vi "control plot scale V1.vi"(6 "offset in":dbl=nan, 7 "action":T2(ring), 8 "Coords":T3, 9 "fraction in":dbl, 11 "plot scale state":T1={"Plot Ref"=refnum, "center"=0.0, "delta"=100.0, "mode"=enum."no filter", "scale cursor index"=0, "history"=100.0, "history array"=[0.5, 0.5, 0.5, 0.5, 0.5, 0.5, 0.5, 0.5, 0.5, 0.5, 0.5, 0.5, 0.5, 0.5, 0.5, 0.5, 0.5, 0.5, 0.5, 0.5, 0.5, 0.5, 0.5, 0.5, 0.5, 0.5, 0.5, 0.5, 0.5, 0.5, 0.5, 0.5, 0.5, 0.5, 0.5, 0.5, 0.5, 0.5, 0.5, 0.5, 0.5, 0.5, 0.5, 0.5, 0.5, 0.5, 0.5, 0.5, 0.5, 0.5, 0.5, 0.5, 0.5, 0.5, 0.5, 0.5, 0.5, 0.5, 0.5, 0.5, 0.5, 0.5, 0.5, 0.5, 0.5, 0.5, 0.5, 0.5, 0.5, 0.5, 0.5, 0.5, 0.5, 0.5, 0.5, 0.5, 0.5, 0.5, 0.5, 0.5, 0.5, 0.5, 0.5, 0.5, 0.5, 0.5, 0.5, 0.5, 0.5, 0.5, 0.5, 0.5, 0.5, 0.5, 0.5, 0.5, 0.5, 0.5, 0.5, 0.5]}) -> (1 "fraction out":dbl, 3 "plot scale state out":T1={"Plot Ref"=refnum, "center"=0.0, "delta"=100.0, "mode"=enum."no filter", "scale cursor index"=0, "history"=100.0, "history array"=[0.5, 0.5, 0.5, 0.5, 0.5, 0.5, 0.5, 0.5, 0.5, 0.5, 0.5, 0.5, 0.5, 0.5, 0.5, 0.5, 0.5, 0.5, 0.5, 0.5, 0.5, 0.5, 0.5, 0.5, 0.5, 0.5, 0.5, 0.5, 0.5, 0.5, 0.5, 0.5, 0.5, 0.5, 0.5, 0.5, 0.5, 0.5, 0.5, 0.5, 0.5, 0.5, 0.5, 0.5, 0.5, 0.5, 0.5, 0.5, 0.5, 0.5, 0.5, 0.5, 0.5, 0.5, 0.5, 0.5, 0.5, 0.5, 0.5, 0.5, 0.5, 0.5, 0.5, 0.5, 0.5, 0.5, 0.5, 0.5, 0.5, 0.5, 0.5, 0.5, 0.5, 0.5, 0.5, 0.5, 0.5, 0.5, 0.5, 0.5, 0.5, 0.5, 0.5, 0.5, 0.5, 0.5, 0.5, 0.5, 0.5, 0.5, 0.5, 0.5, 0.5, 0.5, 0.5, 0.5, 0.5, 0.5, 0.5, 0.5]})   [LabVIEW 2015]
uses:
  <vilib>/Utility/miscctls.llb/LVPoint32TypeDef.ctl
  plot scale state.ctl
  <vilib>/Analysis/6fits.llb/Curve Fitting Criteria.ctl
  <vilib>/Analysis/NI_AALPro.lvlib
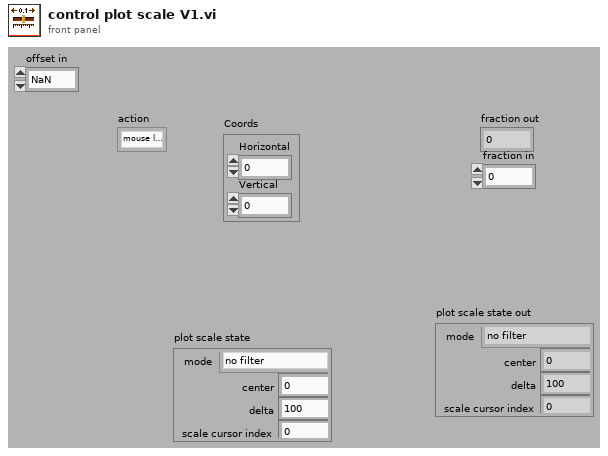
[diagram p1: front panel]
types:
  T1 = typedef "plot scale state.ctl" = cluster{"Plot Ref":refnum<vi>, "center":dbl, "delta":dbl, "mode":enum16{"no filter", "median", "liner fit on median"}, "scale cursor index":i32, "history":dbl, "history array":dbl[]}
  T2 = enum16{"mouse leave", "mouse enter", "mouse move", "manual zoom both", "manual zoom x", "manual zoom y"}
  T3 = typedef "LVPoint32TypeDef.ctl" = cluster{"Horizontal":i32, "Vertical":i32}
  T4 = typedef "LVCursorListTypeDef.ctl" = cluster{"Name":string, "Color":u32, "Style":u8, "Point Style":u8, "Name Visible":bool, "Allow Drag":bool, "Cursor Mode":u32, "Plot":i32, "Index":i32, "Position":cluster{"X":dbl, "Y":dbl}, "X Scale":u32, "Y Scale":u32, "Watch Plots":i32[], "Watch All Plots":bool, "Plot Area":i32, "Label Offset":cluster{"X":dbl, "Y":dbl}}[]
  T5 = cluster{"Name":string, "Color":u32, "Style":u8, "Point Style":u8, "Name Visible":bool, "Allow Drag":bool, "Cursor Mode":u32, "Plot":i32, "Index":i32, "Position":cluster{"X":dbl, "Y":dbl}, "X Scale":u32, "Y Scale":u32, "Watch Plots":i32[], "Watch All Plots":bool, "Plot Area":i32, "Label Offset":cluster{"X":dbl, "Y":dbl}}
  T6 = typedef "LVBoundsTypeDef.ctl" = cluster{"Width":u32, "Height":u32}
  T7 = typedef "LVPositionTypeDef.ctl" = cluster{"Left":i32, "Top":i32}
  T8 = typedef "NI_AALPro.lvlib/Curve Fitting Criteria.ctl" = u16
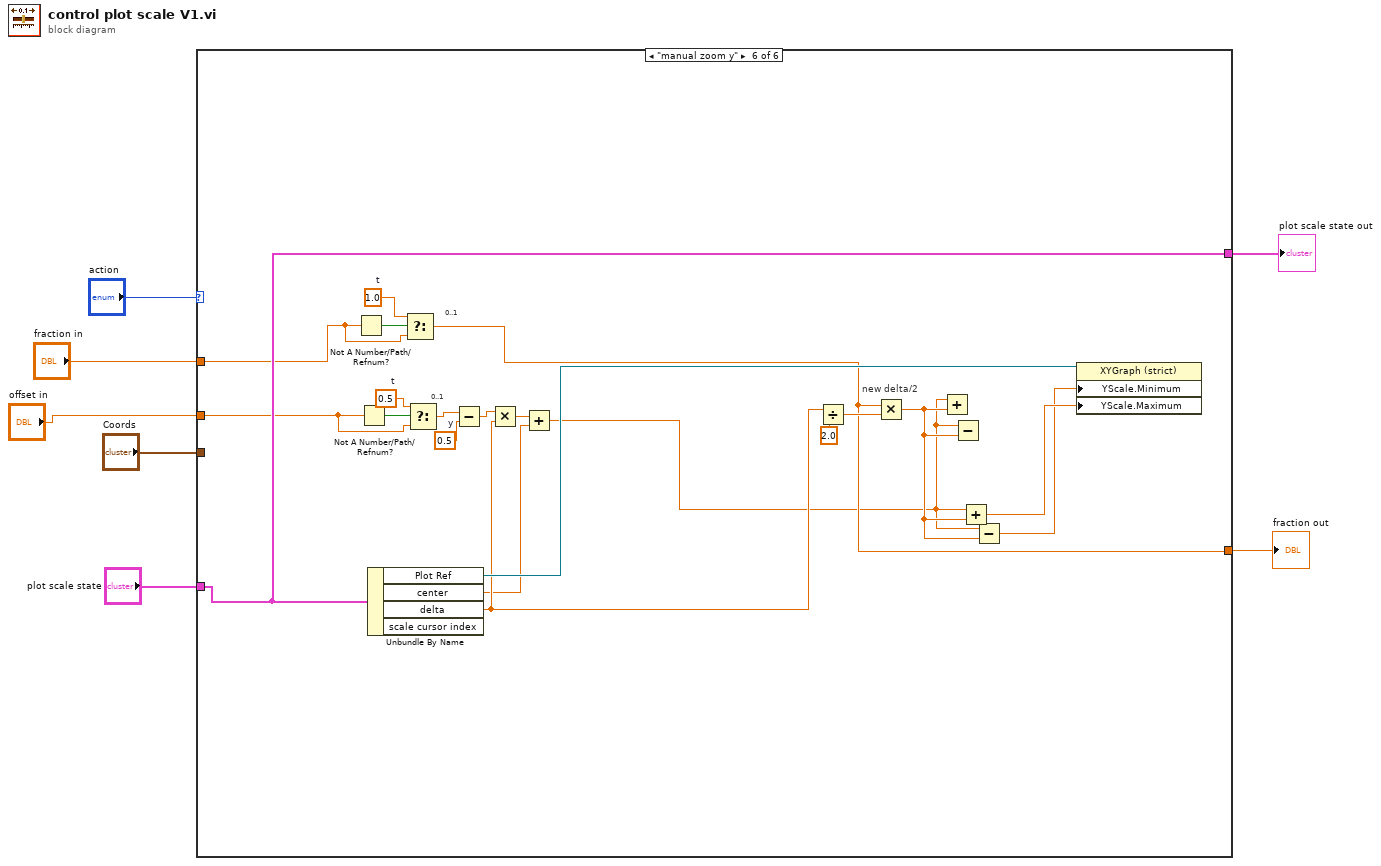
[diagram p0: block diagram]
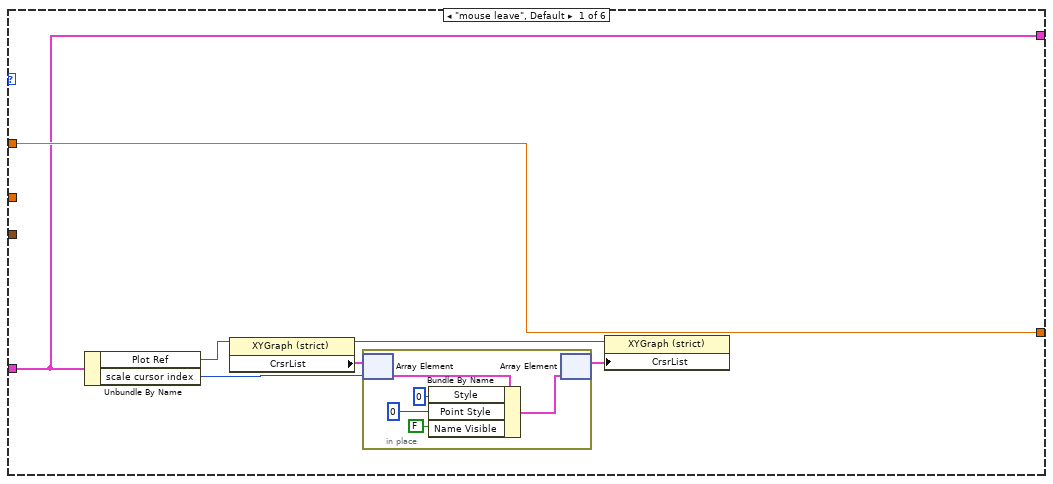
[diagram p2: hidden frame]
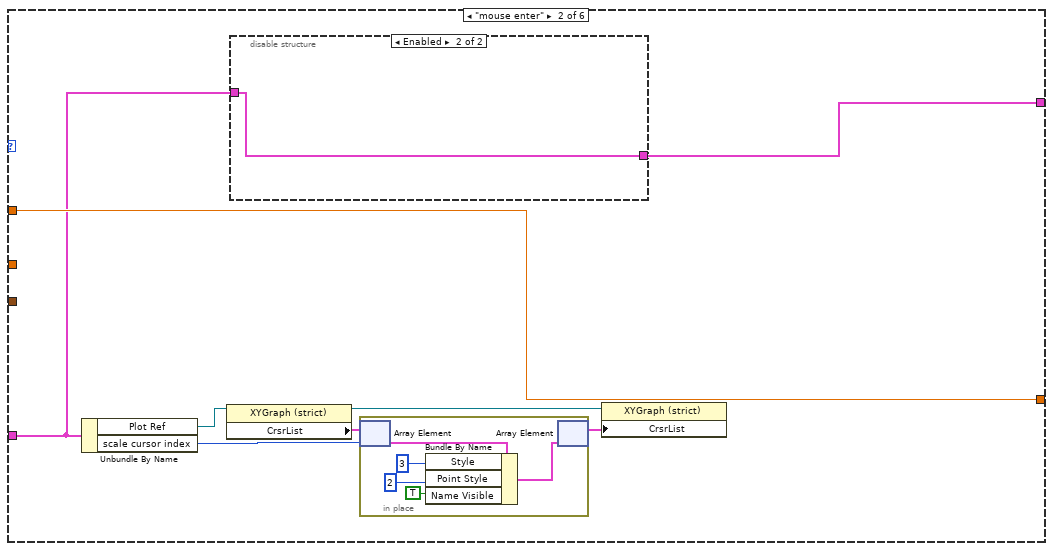
[diagram p3: hidden frame]
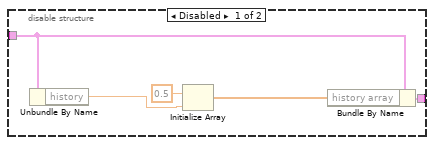
[diagram p4: hidden frame]
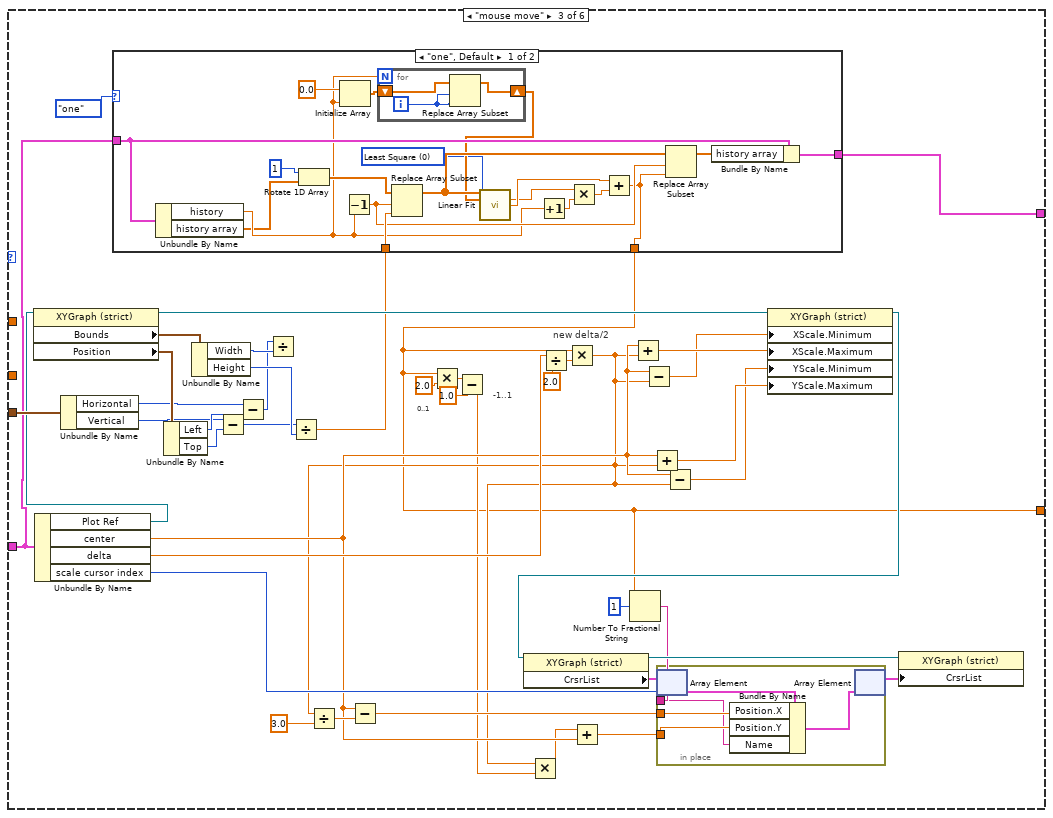
[diagram p5: hidden frame]
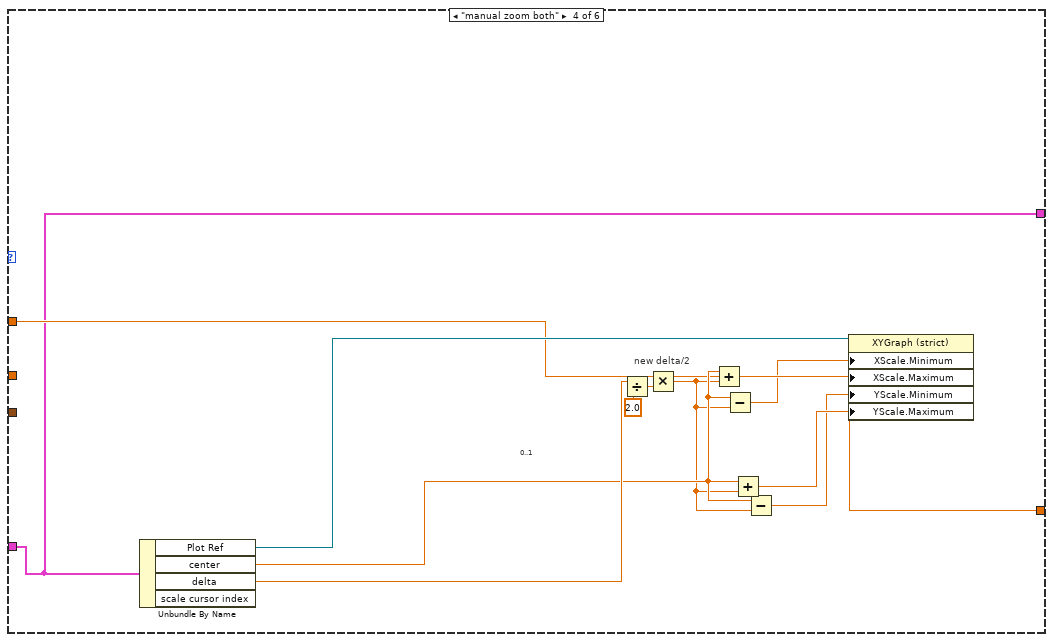
[diagram p7: hidden frame]
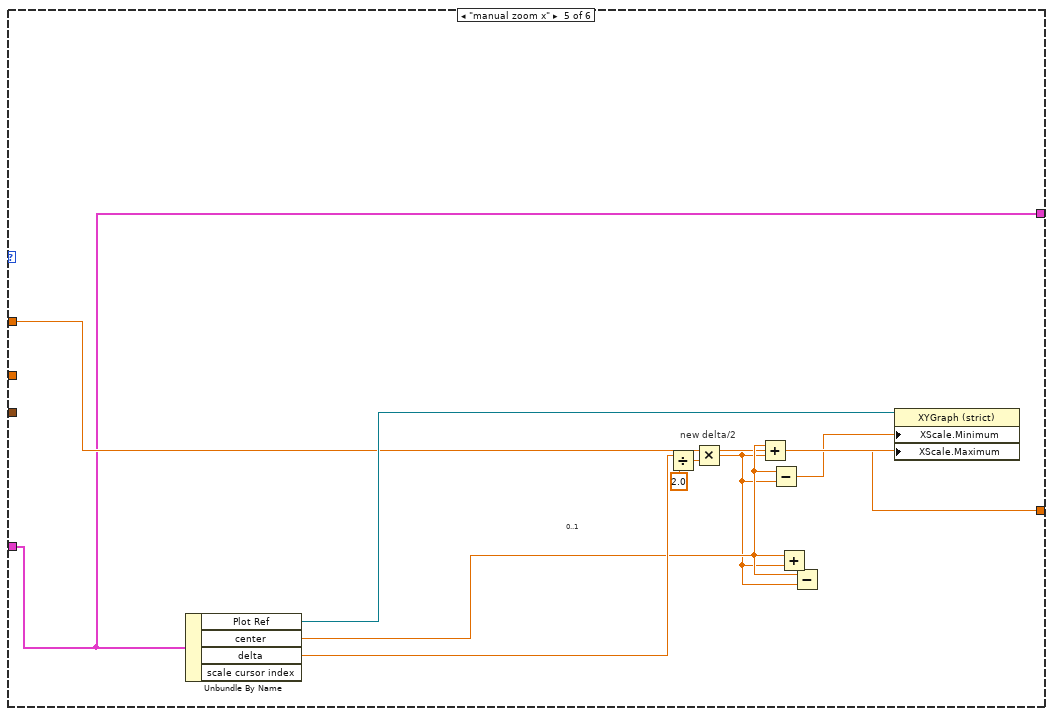
[diagram p8: hidden frame]
diagram:
  n1 = case shown="\"manual zoom y\"" "action" {
    tunnel: "Coords" -> [_ _ w64 _ _ _]
    tunnel: "plot scale state" -> [w8 w21 w43 w111 w123 w147]
    tunnel: [w9 w22 w40 w112 w124 w141] -> w4
    tunnel: "fraction in" -> [w9 w22 _ w112 w124 w142]
    tunnel: [w8 w20 w42 w111 w123 w147] -> w2
    tunnel: "offset in" -> [_ _ _ _ _ w145]
    frame "mouse leave", Default {
      n2 = Unbundle By Name(w8) -> ("Plot Ref"=w14:refnum<vi>, "scale cursor index"=w12:i32)
      n3 = property on="Property Node" class="XYGraph (strict)"(reference=w14) -> (reference out=w10:refnum<vi>, "CrsrList"=w13:T4)  [unwired: 1 in, 1 out]
      n4 = in-place {
        n5 = in-place-array #1(w13, w12) -> (w19:T5)
        n6 = Bundle By Name(cluster=w19, "Style"=u8 0, "Point Style"=u8 0, "Name Visible"=FALSE) -> (w18:T5)
        n7 = in-place-array #1(w18) -> (w11:T4)  [unwired: 1 out]
      }
      n8 = property on="Property Node" class="XYGraph (strict)"(reference=w10, "CrsrList"=w11) -> ()  [unwired: 1 in, 2 out]
    }
    frame "mouse enter" {
      n9 = Unbundle By Name(w21) -> ("Plot Ref"=w27:refnum<vi>, "scale cursor index"=w25:i32)
      n10 = property on="Property Node" class="XYGraph (strict)"(reference=w27) -> (reference out=w23:refnum<vi>, "CrsrList"=w26:T4)  [unwired: 1 in, 1 out]
      n11 = disable-structure shown="Enabled" {
        disable-tunnel: w21 -> [w30 w33]
        disable-tunnel: [w29 w33] -> w20
        frame Disabled {
          n12 = Unbundle By Name(w30) -> ("history"=w31:dbl)
          n13 = Initialize Array(0.5 ("element"), w31) -> (w28:dbl[])
          n14 = Bundle By Name(cluster=w30, "history array"=w28) -> (w29:T1)
        }
        frame Enabled {
        }
      }
      n15 = in-place {
        n16 = in-place-array #2(w26, w25) -> (w38:T5)
        n17 = Bundle By Name(cluster=w38, "Style"=u8 3, "Point Style"=u8 2, "Name Visible"=TRUE) -> (w37:T5)
        n18 = in-place-array #2(w37) -> (w24:T4)  [unwired: 1 out]
      }
      n19 = property on="Property Node" class="XYGraph (strict)"(reference=w23, "CrsrList"=w24) -> ()  [unwired: 1 in, 2 out]
    }
    frame "mouse move" {
      # "-1..1"
      # "0..1"
      # "new delta/2"
      n20 = Unbundle By Name(w43) -> ("Plot Ref"=w62:refnum<vi>, "center"=w51:dbl, "delta"=w63:dbl, "scale cursor index"=w58:i32)
      n21 = property on="Property Node" class="XYGraph (strict)"(reference=w62) -> (reference out=w76:refnum<vi>, "Bounds"=w75:T6, "Position"=w81:T7)  [unwired: 1 in, 1 out]
      n22 = Unbundle By Name(w64) -> ("Horizontal"=w80:i32, "Vertical"=w78:i32)
      n23 = Unbundle By Name(w81) -> ("Left"=w79:i32, "Top"=w77:i32)
      n24 = Unbundle By Name(w75) -> ("Width"=w74:u32, "Height"=w73:u32)
      n25 = Subtract(x=w78, y=w77) -> (x-y=w65:i32)
      n26 = Subtract(x=w80, y=w79) -> (x-y=w66:i32)
      n27 = Divide(x=w66, y=w74) -> ()  [unwired: 1 out]
      n28 = Divide(x=w65, y=w73) -> (x/y=w41:dbl)
      n29 = case shown="\"one\", Default" enum16{"one", "two"}."one" {
        tunnel: w43 -> [w88 w105]
        tunnel: [w100 w105] -> w42
        tunnel: w41 -> [w98 w104]
        tunnel: [w82 w104] -> w40
        frame "one", Default {
          w83 = T8 0 items=["Least Square", "Least Absolute Residual", "Bisquare"] ("method")
          n30 = Unbundle By Name(w88) -> ("history"=w87:dbl, "history array"=w86:dbl[])
          n31 = Rotate 1D Array(1:w86, 2:1 ("n")) -> (0:w97:dbl[])
          n32 = Initialize Array(0.0 ("element"), w87) -> (w95:dbl[])
          n33 = Decrement(x=w87) -> (x-1=w89:dbl)
          n34 = for {
            N: w87 -> [_]
            shift-right: [w102] -> w84
            shift-left: w95 -> [w103]
            i -> [w101]
            n35 = Replace Array Subset(array=w103, new element=w101, index=w101) -> (w102:dbl[])
          }
          n36 = Replace Array Subset(array=w97, new element=w98, index=w89) -> (w85:dbl[])
          n37 = call <vilib>:"Linear Fit.vi"("Y"=w85, "X"=w84, "method"=w83) -> ("slope"=w91:dbl, "intercept"=w92:dbl)  [unwired: 8 in, 3 out]
          n38 = Increment(x=w87) -> (x+1=w94:dbl)
          n39 = Multiply(x=w91, y=w94) -> (x*y=w93:dbl)
          n40 = Add(x=w92, y=w93) -> (x+y=w82:dbl)
          n41 = Replace Array Subset(array=w85, new element=w82, index=w89) -> (w90:dbl[])
          n42 = Bundle By Name(cluster=w88, "history array"=w90) -> (w100:T1)
        }
        frame "two" {
        }
      }
      n43 = Multiply(x=w40, y=2.0) -> (x*y=w53:dbl)
      n44 = Subtract(x=w53, y=1.0) -> (x-y=w46:dbl)
      n45 = Divide(x=w63, y=2.0) -> (x/y=w71:dbl)
      n46 = Multiply(x=w40, y=w71) -> (x*y=w48:dbl)
      n47 = Divide(x=w48, y=3.0) -> (x/y=w55:dbl)
      n48 = Subtract(x=w51, y=w55) -> (x-y=w54:dbl)
      n49 = Multiply(x=w48, y=w46) -> (x*y=w50:dbl)
      n50 = Add(x=w50, y=w51) -> (x+y=w49:dbl)
      n51 = Number To Fractional String(number=w40, width (-)=i16 1) -> (F-format string=w44:string)  [unwired: 2 in]
      n52 = Add(x=w51, y=w48) -> (x+y=w70:dbl)
      n53 = Subtract(x=w51, y=w48) -> (x-y=w69:dbl)
      n54 = Add(x=w51, y=w48) -> (x+y=w68:dbl)
      n55 = Subtract(x=w51, y=w48) -> (x-y=w67:dbl)
      n56 = property on="Property Node" class="XYGraph (strict)"(reference=w76, "XScale.Minimum"=w69, "XScale.Maximum"=w70, "YScale.Minimum"=w67, "YScale.Maximum"=w68) -> (reference out=w57:refnum<vi>)  [unwired: 1 in, 1 out]
      n57 = property on="Property Node" class="XYGraph (strict)"(reference=w57) -> (reference out=w59:refnum<vi>, "CrsrList"=w61:T4)  [unwired: 1 in, 1 out]
      n58 = in-place {
        in-place-border: w54 -> [w108]
        in-place-border: w49 -> [w107]
        in-place-border: w44 -> [w106]
        n59 = in-place-array #3(w61, w58) -> (w110:T5)
        n60 = Bundle By Name(cluster=w110, "Position.X"=w108, "Position.Y"=w107, "Name"=w106) -> (w109:T5)
        n61 = in-place-array #3(w109) -> (w60:T4)  [unwired: 1 out]
      }
      n62 = property on="Property Node" class="XYGraph (strict)"(reference=w59, "CrsrList"=w60) -> ()  [unwired: 1 in, 2 out]
    }
    frame "manual zoom both" {
      # "0..1"
      # "new delta/2"
      n63 = Unbundle By Name(w111) -> ("Plot Ref"=w113:refnum<vi>, "center"=w115:dbl, "delta"=w116:dbl)  [unwired: 1 out]
      n64 = Divide(x=w116, y=2.0) -> (x/y=w121:dbl)
      n65 = Multiply(x=w112, y=w121) -> (x*y=w114:dbl)
      n66 = Add(x=w115, y=w114) -> (x+y=w120:dbl)
      n67 = Subtract(x=w115, y=w114) -> (x-y=w119:dbl)
      n68 = Add(x=w115, y=w114) -> (x+y=w118:dbl)
      n69 = Subtract(x=w115, y=w114) -> (x-y=w117:dbl)
      n70 = property on="Property Node" class="XYGraph (strict)"(reference=w113, "XScale.Minimum"=w119, "XScale.Maximum"=w120, "YScale.Minimum"=w117, "YScale.Maximum"=w118) -> ()  [unwired: 1 in, 2 out]
    }
    frame "manual zoom x" {
      # "0..1"
      # "new delta/2"
      n71 = Unbundle By Name(w123) -> ("Plot Ref"=w125:refnum<vi>, "center"=w127:dbl, "delta"=w128:dbl)  [unwired: 1 out]
      n72 = Divide(x=w128, y=2.0) -> (x/y=w131:dbl)
      n73 = Multiply(x=w124, y=w131) -> (x*y=w126:dbl)
      n74 = Add(x=w127, y=w126) -> (x+y=w130:dbl)
      n75 = Subtract(x=w127, y=w126) -> (x-y=w129:dbl)
      n76 = Add(x=w127, y=w126) -> ()  [unwired: 1 out]
      n77 = Subtract(x=w127, y=w126) -> ()  [unwired: 1 out]
      n78 = property on="Property Node" class="XYGraph (strict)"(reference=w125, "XScale.Minimum"=w129, "XScale.Maximum"=w130) -> ()  [unwired: 1 in, 2 out]
    }
    frame "manual zoom y" {
      w138 = 0.5  # y
      w140 = 0.5  # t
      w143 = 1.0  # t
      # "0..1"
      # "0..1"
      # "new delta/2"
      n79 = Not A Number/Path/Refnum?(number/path/refnum=w142) -> (NaN/Path/Refnum?=w144:bool)
      n80 = Not A Number/Path/Refnum?(number/path/refnum=w145) -> (NaN/Path/Refnum?=w146:bool)
      n81 = Unbundle By Name(w147) -> ("Plot Ref"=w148:refnum<vi>, "center"=w135:dbl, "delta"=w137:dbl)  [unwired: 1 out]
      n82 = Select(t=w143, s=w144, f=w142) -> (s? t:f=w141:dbl)
      n83 = Select(t=w140, s=w146, f=w145) -> (s? t:f=w139:dbl)
      n84 = Subtract(x=w139, y=w138) -> (x-y=w136:dbl)
      n85 = Multiply(x=w136, y=w137) -> (x*y=w134:dbl)
      n86 = Add(x=w134, y=w135) -> (x+y=w133:dbl)
      n87 = Divide(x=w137, y=2.0) -> (x/y=w152:dbl)
      n88 = Multiply(x=w141, y=w152) -> (x*y=w149:dbl)
      n89 = Add(x=w133, y=w149) -> ()  [unwired: 1 out]
      n90 = Subtract(x=w133, y=w149) -> ()  [unwired: 1 out]
      n91 = Add(x=w133, y=w149) -> (x+y=w151:dbl)
      n92 = Subtract(x=w133, y=w149) -> (x-y=w150:dbl)
      n93 = property on="Property Node" class="XYGraph (strict)"(reference=w148, "YScale.Minimum"=w150, "YScale.Maximum"=w151) -> ()  [unwired: 1 in, 2 out]
    }
  }
  "fraction out" <- w4
  "plot scale state out" <- w2
